vi "Amplitude.vi"(8 "error in (no error)":errorcluster, 10 "Amplitude":dbl, 11 "Generador in":refnum<class "Generador.lvclass">) -> (0 "error out":errorcluster, 3 "Generador out":refnum<class "Generador.lvclass">)   [LabVIEW 2020, in "Generador señal.lvlib" / "Generador.lvclass"]
uses:
  Generador.lvclass
  Generador.lvclass/Generador.ctl
  ACQ Generador Messages/Amplitude ACQ Msg/Amplitude ACQ Msg.lvclass/Amplitude ACQ Msg.ctl
  <vilib>/ActorFramework/Message Enqueuer/Message Enqueuer.lvclass/Message Enqueuer.ctl
  <vilib>/ActorFramework/Message Enqueuer/Enqueue.vi
  ACQ Generador Messages/Amplitude ACQ Msg/Amplitude ACQ Msg.lvclass
  C:/Program Files (x86)/National Instruments/LabVIEW 2020/vi.lib/ActorFramework/Message/Message.lvclass
  <vilib>/ActorFramework/Message Priority Queue/Priority Enqueue.vi
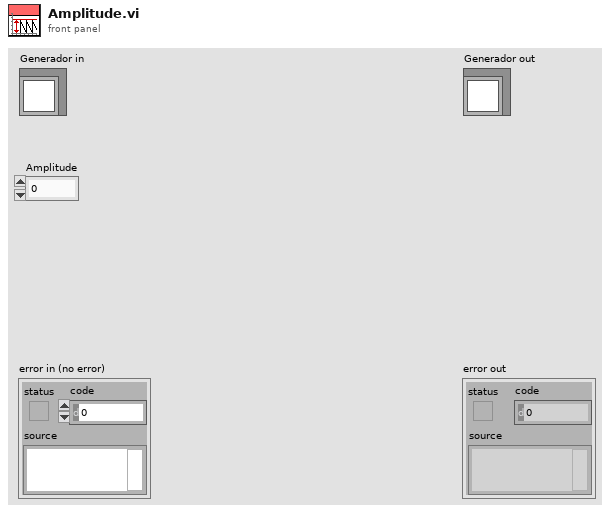
[diagram p1: front panel]
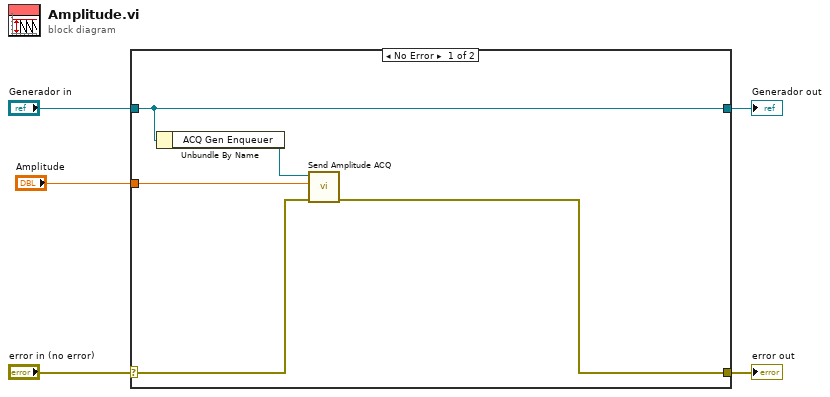
[diagram p0: block diagram]
diagram:
  n1 = case shown="No Error" "error in (no error)" {
    selector: "error in (no error)" -> [w7 w12]
    tunnel: [w6 w12] -> w4
    tunnel: [w10 w11] -> w2
    tunnel: "Generador in" -> [w10 w11]
    tunnel: "Amplitude" -> [w9 _]
    frame No Error {
      n2 = Unbundle By Name(w10) -> ("ACQ Gen Enqueuer"=w8:refnum<class "Message Enqueuer.lvclass">)
      n3 = call "Send Amplitude ACQ.vi"("error in (no error)"=w7, "Amplitude"=w9, "Message Enqueuer"=w8) -> ("error out"=w6:errorcluster)  [unwired: 7 in, 1 out]
    }
    frame Error {
    }
  }
  "error out" <- w4
  "Generador out" <- w2
